vi "Uart read.vi"(0 "RedPitaya connection in":refnum<k5>, 1 "timeout ms (2000)":i32=2000, 5 "Len":u8, 11 "error in":errorcluster) -> (4 "RedPitaya connection out":refnum<k5>, 6 "Raw data out":string, 8 "Output string":string, 15 "error out":errorcluster)   [LabVIEW 2021]
uses:
  Red_Pitaya/RedPitaya.lvlib
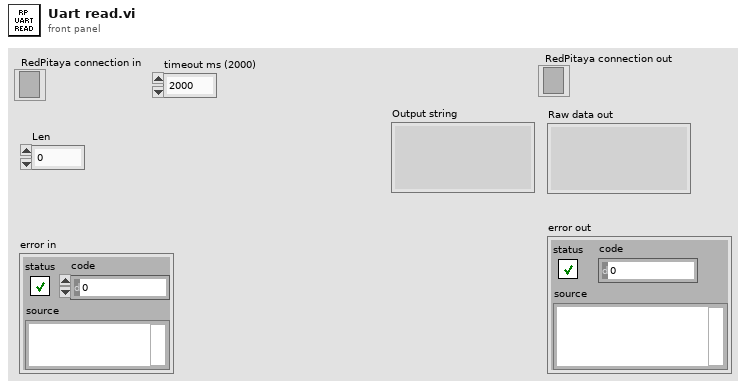
[diagram p1: front panel]
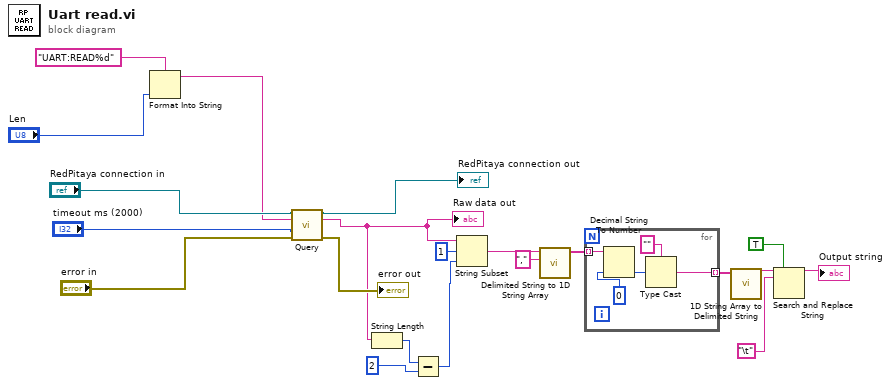
[diagram p0: block diagram]
diagram:
  n1 = Format Into String(format string="UART:READ%d" ("SCPI Query"), "Len") -> (resulting string=w16:string)  [unwired: 2 in, 1 out]
  n2 = call "Query.vi"("RedPitaya connection in"="RedPitaya connection in", "SCPI Query"=w16, "timeout ms (2000)"="timeout ms (2000)", "error in"="error in") -> ("RedPitaya connection out"=→"RedPitaya connection out":refnum<k5>, "data out"=w3:string, "error out"=→"error out":errorcluster)  [unwired: 9 in]
  "Raw data out" <- w3
  n3 = String Length(string=w3) -> (length=w8:i32)
  n4 = Subtract(x=w8, y=u8 2) -> (x-y=w13:i32)
  n5 = String Subset(string=w3, offset (0)=1, length (rest)=w13) -> (substring=w12:string)
  n6 = call <vilib>:"Delimited String to 1D String Array.vi"("delimiter"=",", "delimited string"=w12) -> ("string array"=w10:string[])  [unwired: 9 in]
  n7 = for {
    tunnel: w10 -> [w26] mode=indexing
    tunnel: [w23] -> w9 mode=indexing
    n8 = Decimal String To Number(string=w26, default (0L)=u8 0) -> (number=w25:u8)  [unwired: 1 in, 1 out]
    n9 = Type Cast(type="" ("delimiter"), x=w25) -> (*(type *) &x=w23:string)
  }
  n10 = call <vilib>:"1D String Array to Delimited String.vi"("string array"=w9) -> ("delimited string"=w7:string)  [unwired: 10 in]
  n11 = Search and Replace String(replace all?=TRUE ("replace all? (F)"), input string=w7, search string="\t") -> (result string=→"Output string":string)  [unwired: 5 in, 3 out]
